vi "SET DO AO PLC 3.vi"(10 "USCITE PLC":T1, 11 "Queue":string="PLC_Q") -> ()   [LabVIEW 2019]
uses:
  Uscite PLC 3.ctl
  controls/statoAO_plc_3.ctl
  StatoDO_PLC_3.ctl
  TypeDef_PLC_Q.ctl
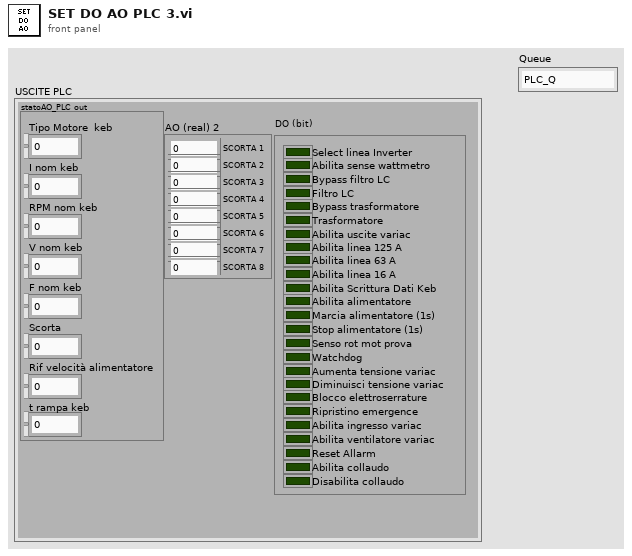
[diagram p1: front panel]
types:
  T1 = typedef "Uscite PLC 3.ctl" = cluster{"AO (real) 2":cluster{"SCORTA 1":dbl, "SCORTA 2":dbl, "SCORTA 3":dbl, "SCORTA 4":dbl, "SCORTA 5":dbl, "SCORTA 6":dbl, "SCORTA 7":dbl, "SCORTA 8":dbl}, "statoAO_PLC out":T2, "DO (bit)":T3}
  T2 = typedef "statoAO_plc_3.ctl" = cluster{"Rif velocità alimentatore":dbl, "Scorta":dbl, "Tipo Motore  keb":dbl, "I nom keb":dbl, "RPM nom keb":dbl, "V nom keb":dbl, "F nom keb":dbl, "t rampa keb":dbl}
  T3 = typedef "StatoDO_PLC_3.ctl" = cluster{"Select linea Inverter":bool, "Abilita sense wattmetro":bool, "Bypass filtro LC":bool, "Filtro LC":bool, "Bypass trasformatore":bool, "Trasformatore":bool, "Abilita uscite variac":bool, "Abilita linea 125 A":bool, "Abilita linea 63 A":bool, "Abilita linea 16 A":bool, "Abilita Scrittura Dati Keb":bool, "Abilita alimentatore":bool, "Marcia alimentatore (1s)":bool, "Stop alimentatore (1s)":bool, "Senso rot mot prova":bool, "Watchdog":bool, "Aumenta tensione variac":bool, "Diminuisci tensione variac ":bool, "Blocco elettroserrature":bool, "Ripristino emergence":bool, "Abilita ingresso variac":bool, "Abilita ventilatore variac":bool, "Reset Allarm":bool, "Scorta 1":bool, "Scorta 2":bool, "Scorta 3":bool, "Scorta 4":bool, "Scorta 5":bool, "Scorta 6":bool, "Scorta 7":bool, "Scorta 8":bool, "Scorta 9":bool, "Abilita collaudo":bool, "Disabilita collaudo ":bool, "Scorta 10":bool, "Scorta 11":bool, "Scorta 12":bool, "Scorta 13":bool, "Scorta 14":bool, "Scorta 15":bool}
  T4 = typedef "TypeDef_PLC_Q.ctl" = cluster{"Message":string, "Data":variant}
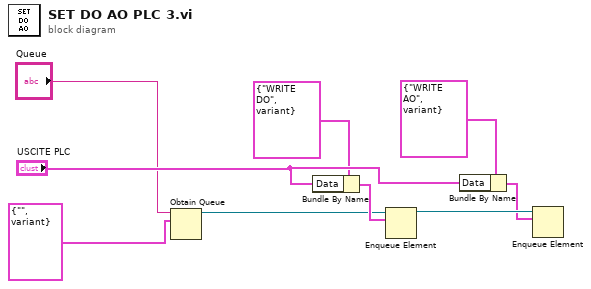
[diagram p0: block diagram]
diagram:
  n1 = Obtain Queue(name (unnamed)="Queue", element data type=T4 {"Message"="", "Data"=variant}) -> (queue out=w2:refnum<queue>)  [unwired: 3 in, 2 out]
  n2 = Bundle By Name(cluster=T4 {"Message"="WRITE DO", "Data"=variant}, "Data"="USCITE PLC") -> (w4:T4)
  n3 = Enqueue Element(queue=w2, element=w4) -> (queue out=w8:refnum<queue>)  [unwired: 2 in, 2 out]
  n4 = Bundle By Name(cluster=T4 {"Message"="WRITE AO", "Data"=variant}, "Data"="USCITE PLC") -> (w7:T4)
  n5 = Enqueue Element(queue=w8, element=w7) -> ()  [unwired: 2 in, 3 out]
